vi "UpdateChannelStatus.vi"(8 "error in (no error)":errorcluster, 9 "Channel Status":string, 10 "Channel Name":string, 11 "Waveforms in":waveform(sgl)[](array[waveform])) -> (0 "error out":errorcluster, 3 "Waveforms out":waveform(sgl)[](array[waveform]))   [LabVIEW 2017, in "McsaAnalysisLowRate.lvlib"]
uses:
  <vilib>/addons/InsightCM/Devices/Shared/Mcsa/McsaAnalysisLowRate/McsaAnalysisLowRate.lvlib
  <vilib>/addons/InsightCM/Utilities/ChannelStatus/ChannelStatus.lvlib
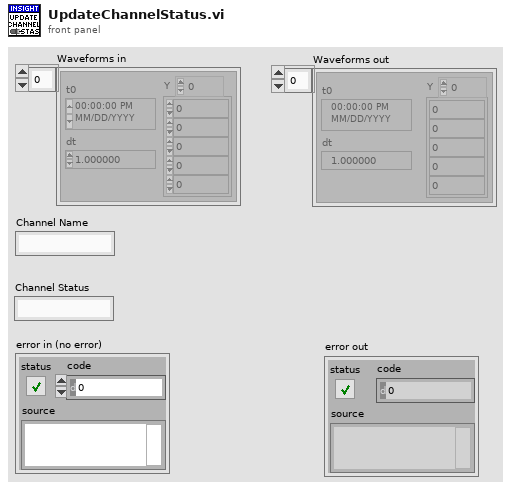
[diagram p1: front panel]
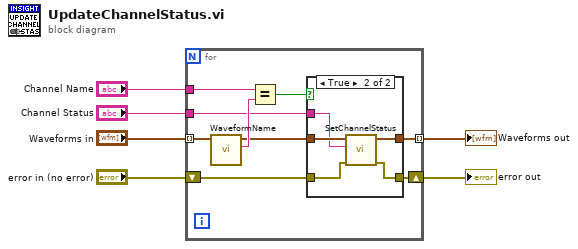
[diagram p0: block diagram]
diagram:
  n1 = for {
    tunnel: "Channel Name" -> [w15]
    tunnel: "Waveforms in" -> [w13] mode=indexing
    tunnel: "Channel Status" -> [w11]
    tunnel: [w10] -> w3 mode=indexing
    shift-right: [w8] -> w1
    shift-left: "error in (no error)" -> [w9]
    n2 = call <vilib>:"WaveformName.vi"("signal in"=w13) -> ("name"=w14:string, "signal out"=w12:waveform(sgl))  [unwired: 9 in]
    n3 = Equal?(x=w15, y=w14) -> (x = y?=w7:bool)
    n4 = case shown="True" w7 {
      tunnel: w12 -> [w17 w22]
      tunnel: w11 -> [_ w21]
      tunnel: [w17 w20] -> w10
      tunnel: w9 -> [w16 w19]
      tunnel: [w16 w18] -> w8
      frame False {
      }
      frame True {
        n5 = call <vilib>:"SetChannelStatus.vi"("error in (no error)"=w19, "Channel Status"=w21, "Waveform in"=w22) -> ("error out"=w18:errorcluster, "Waveform out"=w20:waveform(sgl))  [unwired: 7 in]
      }
    }
  }
  "Waveforms out" <- w3
  "error out" <- w1
